vi "LiDARSteering.vi"() -> ()   [LabVIEW 2024]
uses:
  e33ea129-5426-40bd-9da2-e127971607b1.vi
  <vilib>/Instr/_visa.llb/VISA Configure Serial Port (Instr).vi
  <vilib>/Python/Open Venv Python Session.vi
panel:
  out "Input_Spd(cmd)":dbl=538.4742241275792
  in  "GoBack":bool
  in  "InputSteer(cmd)":dbl=28.559259641865033
  in  "HLV_Gear":u8
  out "PointCloud":T1(graph)=[{"appended array"=[700.0, 700.0, 3500.0, 3500.0, -3500.0, -3500.0, -700.0, -700.0, 700.0], "appended array"=[800.0, -800.0, -800.0, 5200.0, 5200.0, -800.0, -800.0, 800.0, 800.0]}, {"appended array"=[-450.0], "appended array"=[-250.0]}, {"appended array"=[-450.0, -450.0, -800.0, -800.0, 0.0, 0.0, -450.0], "appended array"=[100.0, -800.0, -800.0, 1200.0, 1200.0, 100.0, 100.0]}, {"appended array"=[800.0, 750.0, 800.0, 800.0, 800.0, 800.0, 800.0], "appended array"=[400.0, 350.0, 350.0, 300.0, 250.0, 200.0, 150.0]}, {"appended array"=[450.0, 450.0, 800.0, 800.0, 0.0, 0.0, 450.0], "appended array"=[100.0, -800.0, -800.0, 1200.0, 1200.0, 100.0, 100.0]}, {"appended array"=array[442 elements], "appended array"=array[442 elements]}, {"appended array"=[4.2861222383783204e-13, 0.0], "appended array"=[7000.0, 0.0]}, {"appended array"=[500.0, 500.0, -500.0, -500.0, 500.0], "appended array"=[100.0, 950.0, 950.0, 100.0, 100.0]}]
  in  "격자크기":dbl=50.0
  out "LidarLoop":u32=101
  in  "Ratio_Threshold":i32=4
  in  "min_samples":i32=2
  in  "eps":i32=100
  in  "Spacing":i32=100
  in  "Threshold":i32=2100
  in  "Looking Y":i32=5200
  in  "Looking X":i32=3500
  out "Anthena_Steer":i32
  out "NearSteer":dbl=28.559259641865033
  out "TooClose":bool=TRUE
  out "PythonLoop":u32=101
  in  "LiDAR":refnum<visa-resource-name>="COM5"
  out "VEstop":bool
  in  "length":dbl=1300.0
  out "read buffer":string
  out "Clustering Error":errorcluster
  out "GobackROI":cluster{i32[], i32[]}={[500, 500, -500, -500, 500], [100, 950, 950, 100, 100]}
  in  "Stop":bool
  out "TargetDerection":cluster{dbl[], dbl[]}={[4.2861222383783204e-13, 0.0], [7000.0, 0.0]}
  out "Y_arraysREAL":i32[](array[numeric])=[1650, 1650, 1650, 1650, 1650, 1650, 1650, 1650, 1700, 1700, 1700, 1700, 1700, 1700, 1700, 1700, 1700, 1700, 1700, 1750, 1700]
  out "X_arraysREAL":i32[](array[numeric])=[1000, 1050, 1100, 1150, 1200, 1250, 1300, 1350, 1350, 1400, 1450, 1500, 1550, 1600, 1650, 1700, 1750, 1800, 1850, 1850, 1900]
  out "LookingAt":cluster{i32[], i32[]}={[700, 700, 3500, 3500, -3500, -3500, -700, -700, 700], [800, -800, -800, 5200, 5200, -800, -800, 800, 800]}
  out "NearCarPointsRight":cluster{"ROI_IN_X":dbl[], "ROI_IN_Y":dbl[]}={"ROI_IN_X"=[750.0, 800.0, 800.0, 800.0, 800.0, 800.0], "ROI_IN_Y"=[350.0, 350.0, 300.0, 250.0, 200.0, 150.0]}
  out "NearCarROIRight":cluster{i32[], i32[]}={[450, 450, 800, 800, 0, 0, 450], [100, -800, -800, 1200, 1200, 100, 100]}
  out "Clustered":T2
  out "NearCarROILeft":cluster{i32[], i32[]}={[-450, -450, -800, -800, 0, 0, -450], [100, -800, -800, 1200, 1200, 100, 100]}
  out "NearCarPointsLeft":cluster{"ROI_IN_X":dbl[], "ROI_IN_Y":dbl[]}={"ROI_IN_X"=[-450.0, -550.0], "ROI_IN_Y"=[-250.0, -300.0]}
  out "Y_arrays":dbl[](array[numeric])=[1650.0, 1650.0, 1650.0, 1650.0, 1650.0, 1650.0, 1650.0, 1700.0, 1700.0, 1700.0, 1700.0, 1700.0, 1700.0, 1700.0, 1700.0, 1700.0, 1700.0, 1700.0, 1750.0, 1700.0, 1700.0, 1750.0, 1750.0, 1750.0, 1750.0, 1750.0, 1750.0, 1750.0, 1750.0, 1750.0, 1750.0, 1750.0, 1800.0, 1800.0, 1800.0, 1800.0, 1800.0, 1800.0, 1800.0, 1800.0, 1800.0, 1800.0, 1800.0, 1800.0, 1800.0, 1800.0, 1800.0, 1800.0, 1800.0, 1850.0, 1850.0, 1850.0, 350.0, 350.0, 350.0, 300.0, 250.0, 200.0, 200.0, 150.0, 150.0, 100.0, 50.0, 0.0, -50.0, -100.0, -150.0, -200.0, -250.0, -300.0, -300.0, -350.0, -400.0, -450.0, -500.0, -550.0, -600.0, -650.0, -700.0, -750.0, -800.0, -800.0, -750.0, -750.0, -700.0, -700.0, -650.0, -600.0, -550.0, -550.0, -500.0, -450.0, -400.0, -350.0, -300.0, -250.0, -200.0, -150.0, -100.0, -50.0, 0.0, 50.0, 100.0, 150.0, 200.0, 250.0, 300.0, 350.0, 400.0, 400.0, 450.0, 500.0, 550.0, 600.0, 600.0, 650.0, 650.0, 700.0, 700.0, 750.0, 750.0, 800.0, 800.0, 850.0, 850.0, 900.0, 900.0, 950.0, 950.0, 1000.0, 1000.0, 1050.0, 1050.0, 1100.0, 1100.0, 1150.0, 1150.0, 1200.0, 1200.0, 1250.0, 1250.0, 1300.0, 1300.0, 1350.0, 1400.0, 1450.0, 1500.0, 1550.0, 1600.0, 1650.0, 1700.0, 1750.0, 1800.0, 1850.0, 1900.0, 1950.0, 2000.0, 2050.0, 2100.0, 2150.0, 2200.0, 2250.0, 2300.0, 2350.0, 2400.0, 2450.0, 2500.0, 2550.0, 2600.0, 2600.0, 2650.0, 2700.0, 2750.0, 2800.0, 2850.0, 2900.0, 2950.0, 3000.0, 3050.0, 3100.0, 3150.0, 3200.0, 3250.0, 3300.0, 3350.0, 3400.0, 3450.0, 3450.0, 3500.0, 3550.0, 3600.0, 3650.0, 3700.0, 3750.0, 3800.0, 3850.0, 3900.0, 3950.0, 4000.0, 4000.0, 4100.0, 4150.0, 4200.0, 4250.0, 4300.0, 4350.0, 4400.0, 4450.0, 4500.0, 4550.0, 4600.0, 4650.0, 4700.0, 4750.0, 4800.0, 4900.0, 4950.0, 5000.0, 5050.0, 5100.0, 5150.0, 4500.0, 4500.0, 4600.0, 4550.0, 3800.0, 3700.0, 3650.0, 3600.0, 3550.0, 3500.0, 3500.0, 3450.0, 3400.0, 3350.0, 3300.0, 3250.0, 3250.0, 3200.0, 3150.0, 3200.0, 3200.0, 3200.0, 3400.0, 3450.0, 3200.0, 4700.0, 4700.0, 3700.0, 3450.0, 3400.0, 3450.0, 3500.0, 3500.0, 3450.0, 3400.0, 3400.0, 3350.0, 3300.0, 3300.0, 3250.0, 1600.0, 1600.0, 1650.0, 1600.0, 1650.0, 1735.0877192982457, -160.3448275862069, 1825.7462686567164, 5025.0, 4500.0, 4575.0, 3392.1052631578946, 3425.0, 4700.0, 3395.8333333333335, 1827.3513645224173, 1919.6150097465888, 2011.8786549707602, 2104.142300194932, 2196.4059454191033, 2288.669590643275, 2380.9332358674465, 2473.196881091618, 2565.4605263157896, 2657.7241715399614, 2749.9878167641327, 2842.251461988304, 2934.5151072124754, 3026.778752436647, 3119.042397660819, 3211.3060428849903, 3303.5696881091617, 1824.0304709141276, 1912.9732225300093, 2001.9159741458911, 2090.858725761773, 2179.801477377655, 2268.7442289935366, 2357.6869806094182, 2446.6297322253004, 2535.572483841182, 2624.5152354570637, 2713.457987072946, 2802.400738688827, 2891.343490304709, 2980.2862419205912, 3069.228993536473, 3158.1717451523546, 3247.114496768236, 3336.057248384118, 1817.938596491228, 1900.7894736842106, 1983.640350877193, 2066.4912280701756, 2149.342105263158, 2232.1929824561403, 2315.043859649123, 2397.8947368421054, 2480.745614035088, 2563.59649122807, 2646.4473684210525, 2729.2982456140353, 2812.149122807017, 2895.0, 2977.8508771929824, 3060.7017543859647, 3143.5526315789475, 3226.4035087719294, 3309.254385964912, 4515.0, 4530.0, 4545.0, 4560.0, 4407.675438596491, 4315.350877192983, 4223.026315789473, 4130.701754385965, 4038.377192982456, 3946.0526315789475, 3853.7280701754385, 3761.40350877193, 3669.078947368421, 3576.754385964912, 3484.4298245614036, 4417.307692307692, 4334.615384615385, 4251.923076923077, 4169.2307692307695, 4086.5384615384614, 4003.846153846154, 3921.153846153846, 3838.4615384615386, 3755.769230769231, 3673.076923076923, 3590.3846153846152, 3507.6923076923076, 4588.888888888889, 4602.777777777777, 4616.666666666667, 4630.555555555556, 4644.444444444444, 4658.333333333333, 4672.222222222223, 4686.111111111111, 4479.166666666667, 4383.333333333333, 4287.5, 4191.666666666667, 4095.8333333333335, 4000.0, 3904.166666666667, 3808.3333333333335, 3712.5, 3616.666666666667, 3520.8333333333335, 3403.0701754385964, 3414.035087719298, 3392.6378446115286, 3393.1704260651627, 3393.7030075187968, 3394.2355889724313, 3394.7681704260654, 3395.3007518796994, 3417.7083333333335, 3410.416666666667, 3403.125, 4684.615384615385, 4669.2307692307695, 4653.846153846154, 4638.461538461538, 4623.076923076923, 4607.692307692308, 4592.307692307692, 4576.923076923077, 4561.538461538462, 4546.153846153846, 4530.7692307692305, 4515.384615384615, 4606.8452380952385, 4513.690476190476, 4420.535714285715, 4327.380952380952, 4234.226190476191, 4141.071428571428, 4047.916666666667, 3954.761904761905, 3861.607142857143, 3768.452380952381, 3675.2976190476193, 3582.1428571428573, 3488.9880952380954, 3486.538461538462, 3577.24358974359, 3667.9487179487182, 3758.653846153846, 3849.3589743589746, 3940.0641025641025, 4030.769230769231, 4121.474358974359, 4212.179487179487, 4302.884615384615, 4393.589743589744, 4484.294871794872]
  out "X_arrays":dbl[](array[numeric])=[1050.0, 1100.0, 1150.0, 1200.0, 1250.0, 1300.0, 1350.0, 1350.0, 1400.0, 1450.0, 1500.0, 1550.0, 1600.0, 1650.0, 1700.0, 1750.0, 1800.0, 1850.0, 1850.0, 1900.0, 1950.0, 2000.0, 2050.0, 2100.0, 2150.0, 2200.0, 2250.0, 2300.0, 2350.0, 2400.0, 2450.0, 2500.0, 2500.0, 2550.0, 2600.0, 2650.0, 2700.0, 2750.0, 2800.0, 2850.0, 2900.0, 2950.0, 3000.0, 3050.0, 3100.0, 3150.0, 3200.0, 3250.0, 3300.0, 3350.0, 3400.0, 3450.0, 750.0, 800.0, 850.0, 800.0, 800.0, 800.0, 850.0, 800.0, 850.0, 850.0, 850.0, 850.0, 850.0, 850.0, 850.0, 850.0, 850.0, 850.0, 900.0, 900.0, 900.0, 900.0, 900.0, 900.0, 900.0, 900.0, 900.0, 900.0, 900.0, -2250.0, -2250.0, -2300.0, -2300.0, -2250.0, -2300.0, -2300.0, -2300.0, -2350.0, -2300.0, -2300.0, -2300.0, -2300.0, -2300.0, -2300.0, -2300.0, -2300.0, -2300.0, -2300.0, -2300.0, -2300.0, -2300.0, -2300.0, -2300.0, -2300.0, -2300.0, -2300.0, -2250.0, -2300.0, -2300.0, -2300.0, -2300.0, -2300.0, -2250.0, -2250.0, -2300.0, -2250.0, -2300.0, -2300.0, -2250.0, -2300.0, -2250.0, -2300.0, -2250.0, -2300.0, -2250.0, -2250.0, -2300.0, -2300.0, -2250.0, -2250.0, -2300.0, -2250.0, -2300.0, -2250.0, -2300.0, -2250.0, -2300.0, -2300.0, -2250.0, -2300.0, -2250.0, -2250.0, -2250.0, -2250.0, -2250.0, -2250.0, -2250.0, -2250.0, -2250.0, -2250.0, -2250.0, -2250.0, -2250.0, -2250.0, -2250.0, -2250.0, -2250.0, -2250.0, -2250.0, -2250.0, -2250.0, -2250.0, -2250.0, -2250.0, -2250.0, -2250.0, -2250.0, -2300.0, -2300.0, -2300.0, -2300.0, -2300.0, -2300.0, -2300.0, -2300.0, -2300.0, -2300.0, -2300.0, -2300.0, -2300.0, -2300.0, -2300.0, -2300.0, -2300.0, -2300.0, -2350.0, -2350.0, -2350.0, -2350.0, -2350.0, -2350.0, -2350.0, -2350.0, -2350.0, -2350.0, -2350.0, -2350.0, -2400.0, -2400.0, -2400.0, -2400.0, -2400.0, -2400.0, -2400.0, -2400.0, -2400.0, -2400.0, -2400.0, -2400.0, -2400.0, -2400.0, -2400.0, -2400.0, -2450.0, -2450.0, -2450.0, -2450.0, -2450.0, -2450.0, 650.0, 700.0, 1100.0, 1150.0, 950.0, 950.0, 950.0, 950.0, 950.0, 950.0, 1000.0, 1000.0, 1000.0, 1000.0, 1000.0, 1000.0, 1050.0, 1050.0, 1050.0, 1100.0, 1150.0, 1200.0, 1300.0, 1350.0, 1250.0, 1900.0, 1950.0, 1600.0, 1500.0, 1550.0, 1600.0, 1600.0, 1650.0, 1650.0, 1650.0, 1700.0, 1650.0, 1650.0, 1700.0, 1700.0, 900.0, 950.0, 950.0, 1000.0, 1000.0, 2118.4210526315787, 856.8965517241379, -2300.0, -2450.0, 675.0, 1125.0, 1028.9473684210527, 1325.0, 1925.0, 1633.3333333333333, 2091.4717348927875, 2064.522417153996, 2037.5730994152045, 2010.623781676413, 1983.6744639376216, 1956.7251461988303, 1929.7758284600388, 1902.8265107212474, 1875.877192982456, 1848.9278752436646, 1821.9785575048732, 1795.029239766082, 1768.0799220272904, 1741.130604288499, 1714.1812865497075, 1687.231968810916, 1660.2826510721247, 2076.6620498614957, 2034.9030470914126, 1993.1440443213294, 1951.3850415512463, 1909.6260387811633, 1867.8670360110802, 1826.108033240997, 1784.349030470914, 1742.590027700831, 1700.8310249307478, 1659.0720221606648, 1617.3130193905818, 1575.5540166204987, 1533.7950138504154, 1492.0360110803324, 1450.2770083102494, 1408.5180055401663, 1366.759002770083, 2063.9473684210525, 2009.4736842105262, 1954.9999999999998, 1900.5263157894735, 1846.0526315789473, 1791.5789473684208, 1737.1052631578946, 1682.6315789473683, 1628.157894736842, 1573.6842105263158, 1519.2105263157894, 1464.736842105263, 1410.2631578947367, 1355.7894736842104, 1301.3157894736842, 1246.842105263158, 1192.3684210526317, 1137.8947368421054, 1083.421052631579, 765.0, 855.0, 945.0, 1035.0, 704.4956140350878, 733.9912280701755, 763.4868421052631, 792.9824561403509, 822.4780701754387, 851.9736842105264, 881.469298245614, 910.9649122807018, 940.4605263157896, 969.9561403508773, 999.4517543859649, 725.0, 775.0, 825.0, 875.0, 925.0, 975.0, 1025.0, 1075.0, 1125.0, 1175.0, 1225.0, 1275.0, 1213.888888888889, 1302.7777777777778, 1391.6666666666665, 1480.5555555555557, 1569.4444444444443, 1658.3333333333333, 1747.2222222222222, 1836.111111111111, 1141.6666666666667, 1158.3333333333333, 1175.0, 1191.6666666666667, 1208.3333333333333, 1225.0, 1241.6666666666667, 1258.3333333333333, 1275.0, 1291.6666666666667, 1308.3333333333333, 1127.6315789473686, 1226.3157894736842, 1115.2882205513786, 1201.6290726817042, 1287.96992481203, 1374.310776942356, 1460.6516290726815, 1546.9924812030074, 1402.0833333333333, 1479.1666666666665, 1556.25, 1828.8461538461538, 1732.6923076923076, 1636.5384615384614, 1540.3846153846152, 1444.2307692307693, 1348.076923076923, 1251.9230769230767, 1155.7692307692307, 1059.6153846153848, 963.4615384615385, 867.3076923076922, 771.1538461538462, 1904.1666666666667, 1883.3333333333333, 1862.5, 1841.6666666666667, 1820.8333333333333, 1800.0, 1779.1666666666665, 1758.3333333333333, 1737.5, 1716.6666666666665, 1695.8333333333333, 1675.0, 1654.1666666666665, 1594.230769230769, 1555.128205128205, 1516.0256410256409, 1476.923076923077, 1437.8205128205127, 1398.7179487179487, 1359.6153846153845, 1320.5128205128203, 1281.4102564102564, 1242.3076923076924, 1203.2051282051282, 1164.102564102564]
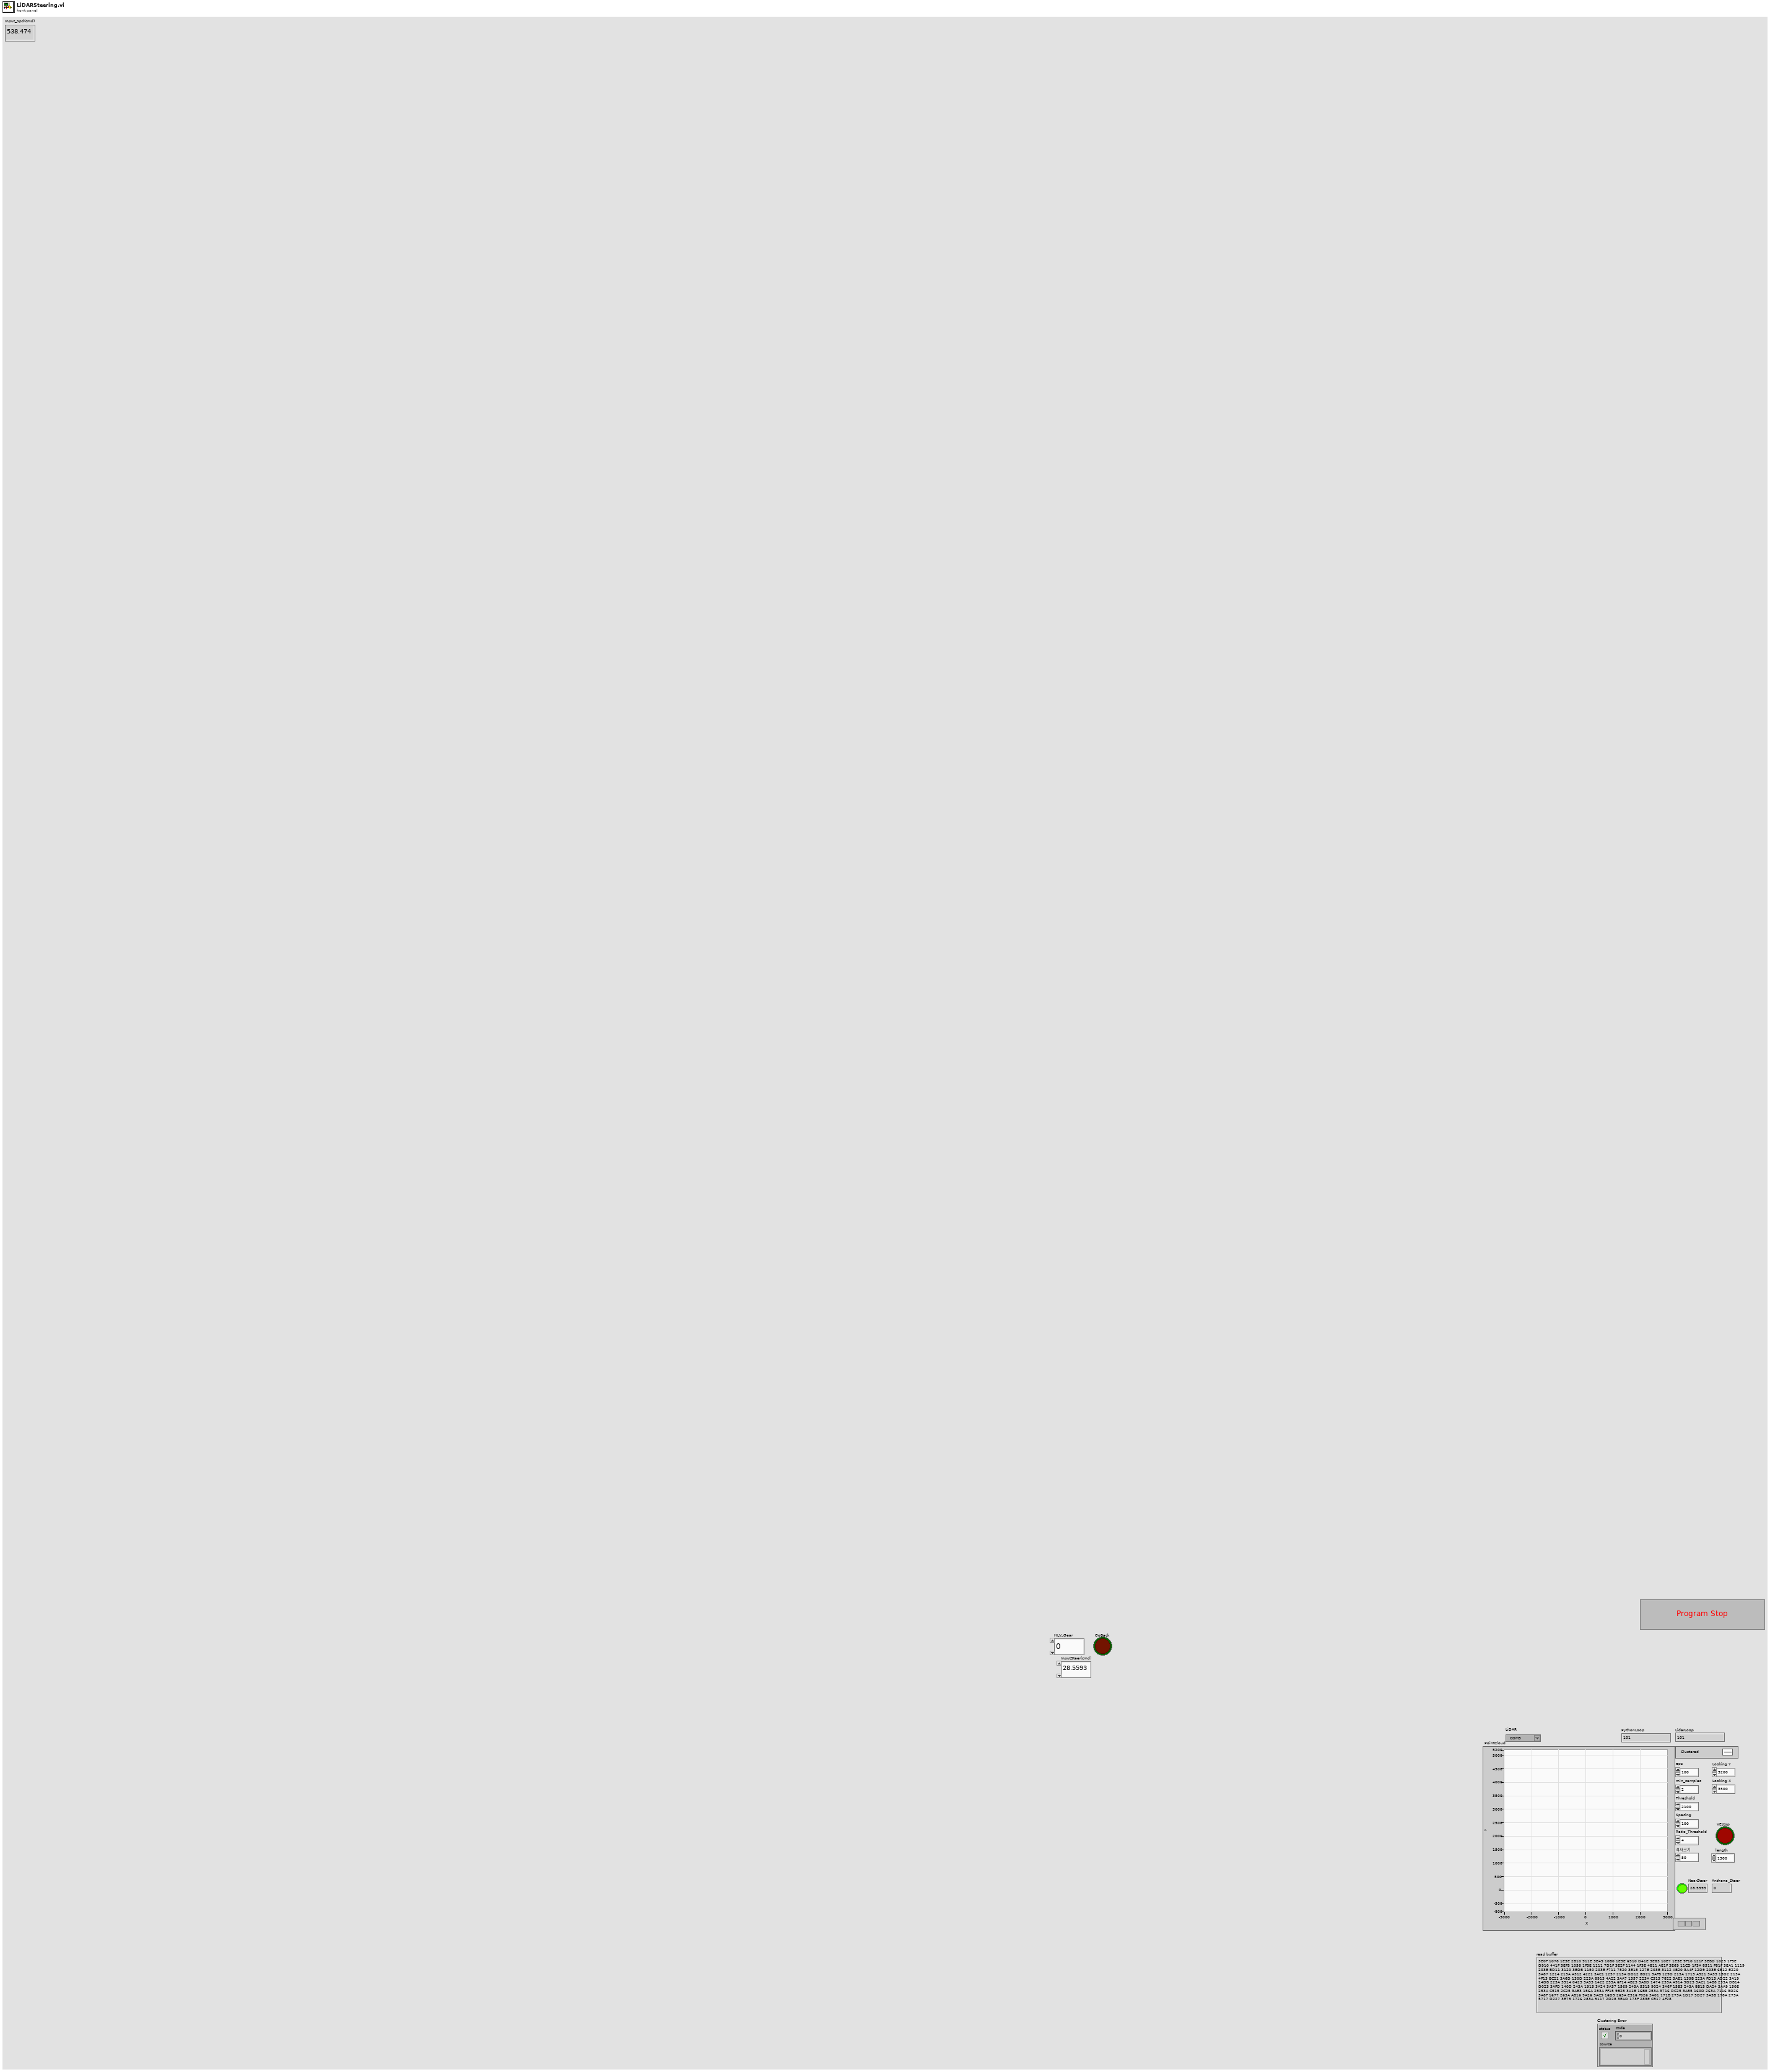
[diagram p1: front panel]
types:
  T1 = cluster{"appended array":dbl[], "appended array":dbl[]}[]
  T2 = cluster{"appended array":dbl[], "appended array":dbl[]}
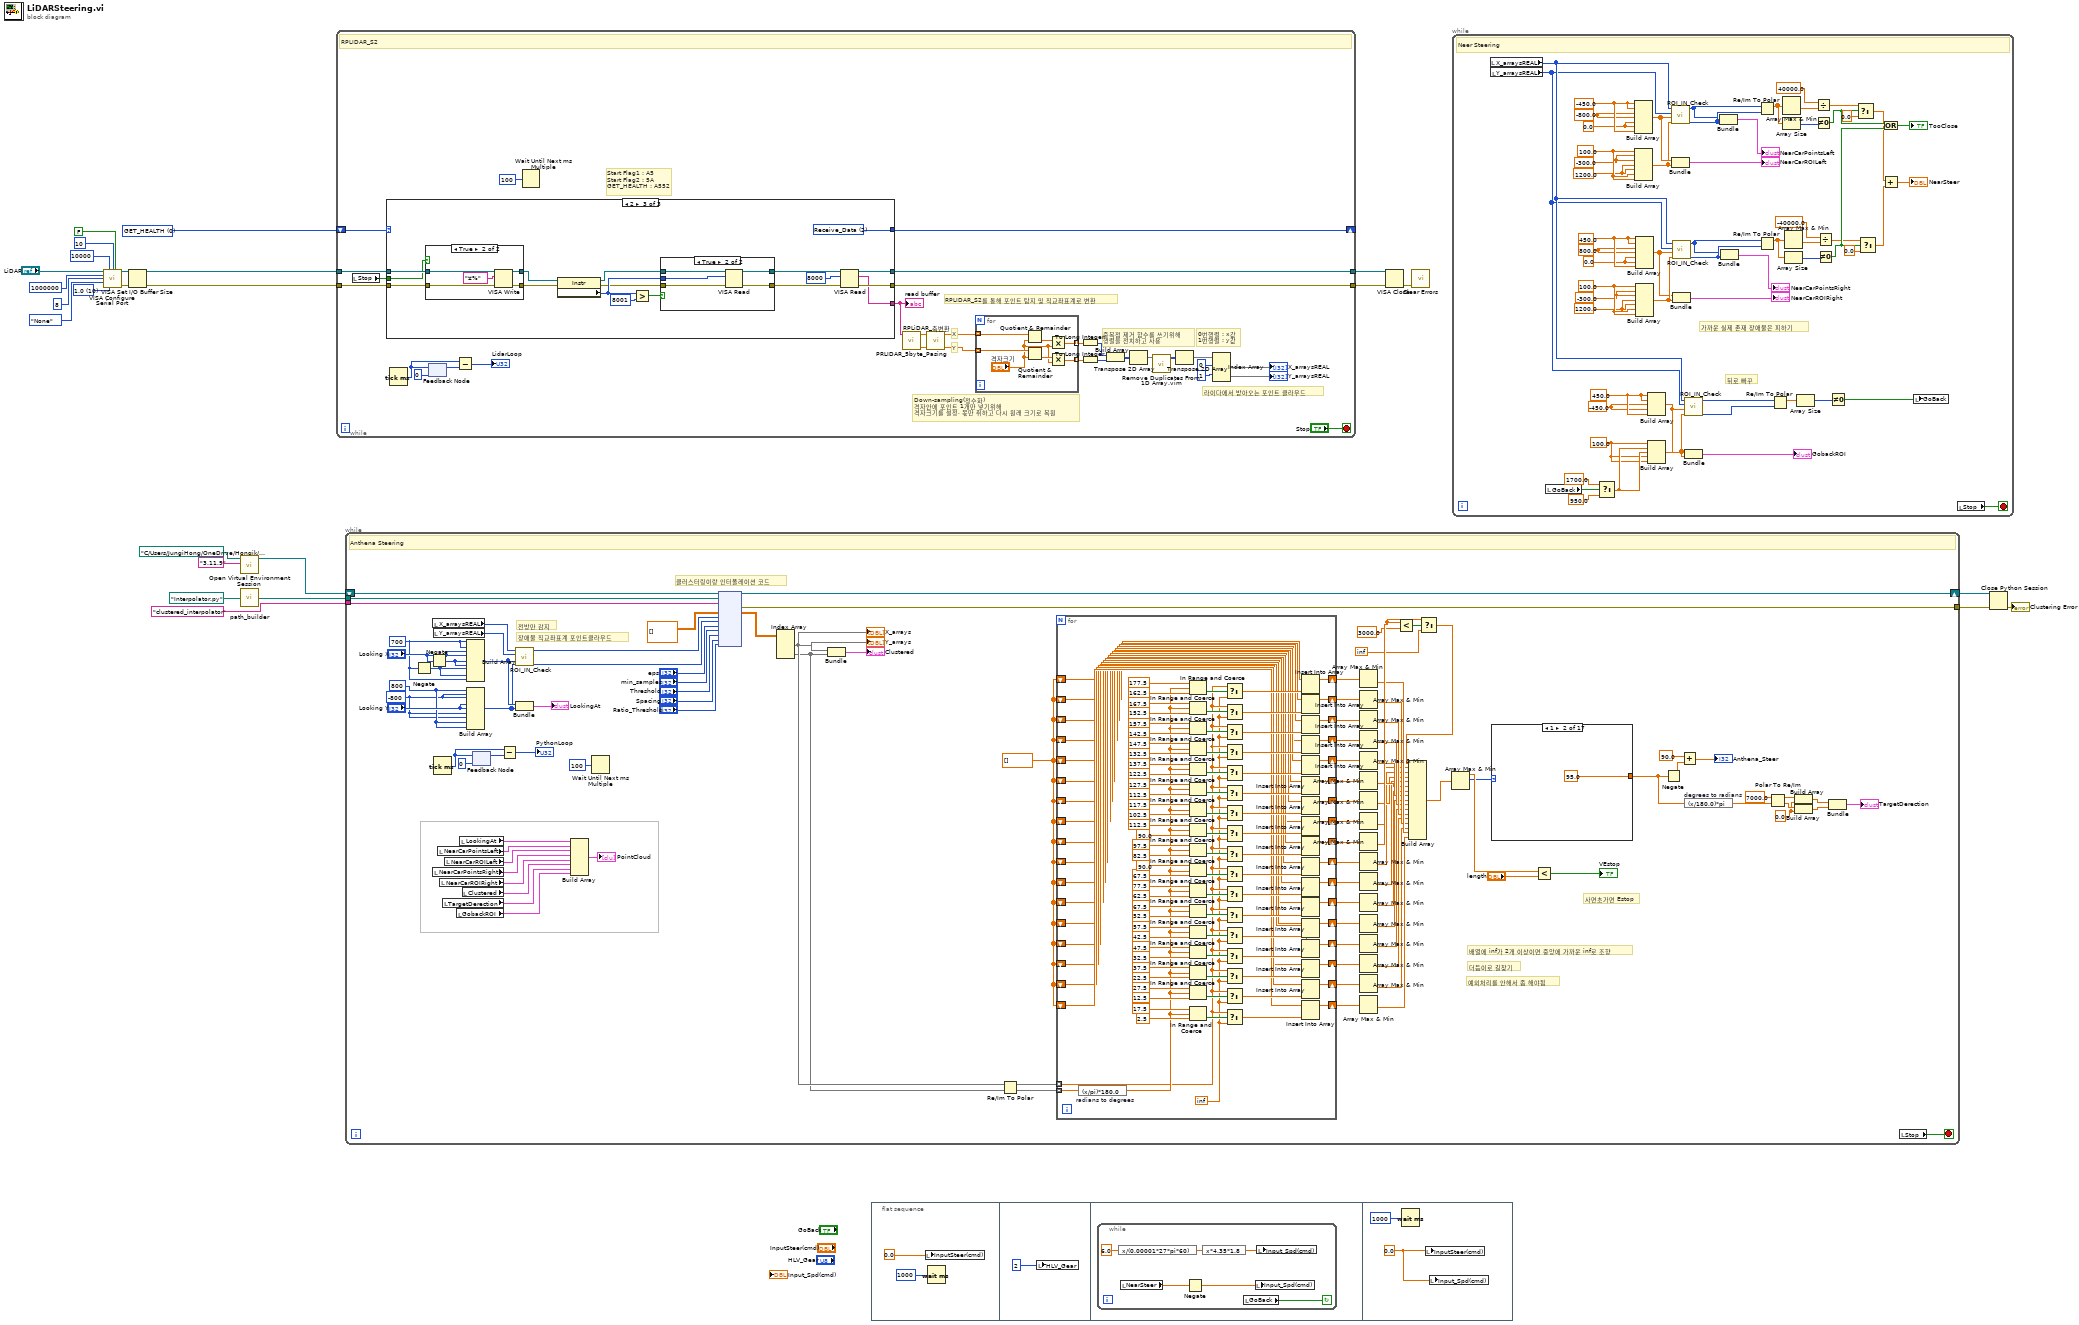
[diagram p0: block diagram]
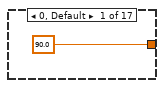
[diagram p2: hidden frame]
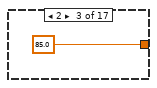
[diagram p3: hidden frame]
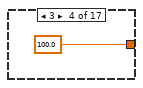
[diagram p4: hidden frame]
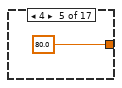
[diagram p5: hidden frame]
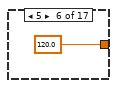
[diagram p6: hidden frame]
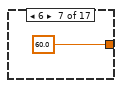
[diagram p7: hidden frame]
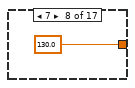
[diagram p8: hidden frame]
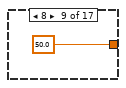
[diagram p9: hidden frame]
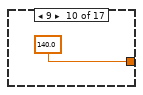
[diagram p10: hidden frame]
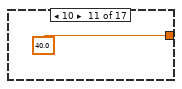
[diagram p11: hidden frame]
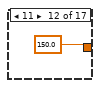
[diagram p12: hidden frame]
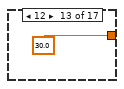
[diagram p13: hidden frame]
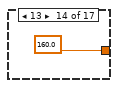
[diagram p14: hidden frame]
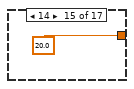
[diagram p15: hidden frame]
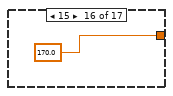
[diagram p16: hidden frame]
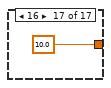
[diagram p17: hidden frame]
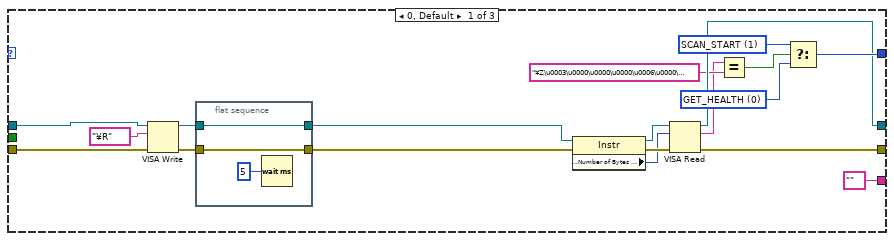
[diagram p18: hidden frame]
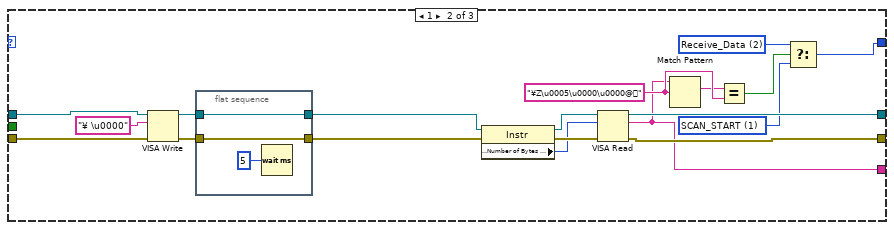
[diagram p19: hidden frame]
diagram:
  w11 = u16 10 items=["1.0"=10, "1.5"=15, "2.0"=20] ("stop bits (10: 1 bit)")
  w13 = u16 0 items=["GET_HEALTH", "SCAN_START", "Receive_Data"]
  n1 = call-poly "VISA Configure Serial Port"("VISA resource name"="LiDAR", "timeout (10sec)"=u32 10000, "termination char\n(0xA = '\\n' = LF)"=u8 10 ("termination char\n(0xA = '\\n' = LF)"), "Enable Termination\nChar (T)"=FALSE ("Enable Termination\nChar (T)"), "baud rate (9600)"=u32 1000000, "data bits (8)"=u16 8, "parity (0:none)"=enum16{"None", "Odd", "Even", "Mark", "Space"}."None", "stop bits (10: 1 bit)"=w11) -> ("VISA resource name out"=w20:refnum<visa-resource-name>, "error out"=w19:errorcluster)  [unwired: 6 in]
  n2 = VISA Set I/O Buffer Size(VISA resource name=w20, error in (no error)=w19) -> (VISA resource name out=w15:refnum<visa-resource-name>, error out=w14:errorcluster)  [unwired: 2 in]
  n3 = call-poly <vilib>:"Open Virtual Environment Session.vi"("Python version"="3.11.9", "Env path"=path "C:/Users/JungiHong/OneDrive/Hongik/HI-RACE/2026-01/.venv" ("Name")) -> ("session out"=w2:refnum<k35>)  [unwired: 8 in, 1 out]
  n4 = call "path_builder.vi"("Name"=path "Interpolator.py") -> ("appended path"=w6:path)
  n5 = while {
    tunnel: [w45] -> w24
    tunnel: [w46] -> w23
    tunnel: w15 -> [w54]
    tunnel: w14 -> [w53]
    shift-right: [w52] -> _
    shift-left: w13 -> [w55]
    stop <- "Stop" stop-if-true
    # "라이다에서 받아오는 포인트 클라우드"
    # "RPLIDAR_S2를 통해 포인트 탐지 및 직교좌표계로 변환"
    # "Start Flag1 : A5\nStart Flag2 : 5A \nGET_HEALTH : A552"
    # "0번행렬 : x값\n1번행렬 : y값"
    # "중복점 제거 함수를 쓰기위해\n행렬을 전치하고 사용"
    # "Down-sampling(정수화)\n격자안에 포인트 1개만 넣기위해\n격자크기를 설정, 몫만 취하고 다시 원래 크기로 복원"
    # "Y"
    # "X"
    # "RPLIDAR_S2"
    n6 = local read "Stop"() -> (w51:bool)
    n7 = case shown="2" w55 {
      tunnel: w54 -> [w80 w98 w121]
      tunnel: w53 -> [w79 w97 w120]
      tunnel: [w81 w94 w107] -> w52
      tunnel: [w70 w95 w123] -> w46
      tunnel: [w69 w96 w122] -> w45
      tunnel: w51 -> [_ _ w119]
      tunnel: ["" ("read buffer") w92 w118] -> w30
      frame 0, Default {
        w63 = u16 0 items=["GET_HEALTH", "SCAN_START", "Receive_Data"]
        w64 = u16 1 items=["GET_HEALTH", "SCAN_START", "Receive_Data"]
        n8 = VISA Write(VISA resource name=w80, write buffer="¥R", error in (no error)=w79) -> (VISA resource name out=w74:refnum<visa-resource-name>, error out=w73:errorcluster)  [unwired: 1 out]
        n9 = flat-sequence {
          tunnel: w74 -> [w83]
          tunnel: w73 -> [w82]
          tunnel: [w83] -> w72
          tunnel: [w82] -> w71
          frame #0 {
            n10 = Wait (ms)(milliseconds to wait=u32 5 ("대기 시간 (ms)")) -> ()  [unwired: 1 out]
          }
        }
        n11 = property class="Instr"(reference=w72, error in=w71) -> (reference out=w77:refnum<visa-resource-name>, error out=w76:errorcluster, "Serial Settings:Number of Bytes at Serial Port"=w75:u32)
        n12 = VISA Read(VISA resource name=w77, byte count=w75, error in (no error)=w76) -> (VISA resource name out=w69:refnum<visa-resource-name>, read buffer=w66:string, error out=w70:errorcluster)  [unwired: 1 out]
        n13 = Equal?(x=w66, y="¥Z\u0003\u0000\u0000\u0000\u0006\u0000\u0000\u0000") -> (x = y?=w67:bool)
        n14 = Select(t=w64, s=w67, f=w63) -> (s? t:f=w81:u16)
      }
      frame 1 {
        w85 = u16 2 items=["GET_HEALTH", "SCAN_START", "Receive_Data"]
        w86 = u16 1 items=["GET_HEALTH", "SCAN_START", "Receive_Data"]
        w99 = "¥Z\u0005\u0000\u0000@"
        n15 = VISA Write(VISA resource name=w98, write buffer="¥ \u0000", error in (no error)=w97) -> (VISA resource name out=w101:refnum<visa-resource-name>, error out=w102:errorcluster)  [unwired: 1 out]
        n16 = flat-sequence {
          tunnel: w101 -> [w105]
          tunnel: w102 -> [w104]
          tunnel: [w105] -> w88
          tunnel: [w104] -> w87
          frame #0 {
            n17 = Wait (ms)(milliseconds to wait=u32 5 ("대기 시간 (ms)")) -> ()  [unwired: 1 out]
          }
        }
        n18 = property class="Instr"(reference=w88, error in=w87) -> (reference out=w91:refnum<visa-resource-name>, error out=w90:errorcluster, "Serial Settings:Number of Bytes at Serial Port"=w89:u32)
        n19 = VISA Read(VISA resource name=w91, byte count=w89, error in (no error)=w90) -> (VISA resource name out=w96:refnum<visa-resource-name>, read buffer=w92:string, error out=w95:errorcluster)  [unwired: 1 out]
        n20 = Match Pattern(string=w92, regular expression=w99) -> (match substring=w93:string)  [unwired: 1 in, 3 out]
        n21 = Equal?(x=w93, y=w99) -> (x = y?=w103:bool)
        n22 = Select(t=w85, s=w103, f=w86) -> (s? t:f=w94:u16)
      }
      frame 2 {
        w107 = u16 2 items=["GET_HEALTH", "SCAN_START", "Receive_Data"]
        n23 = case shown="True" w119 {
          tunnel: w121 -> [w132 w136]
          tunnel: w120 -> [w131 w135]
          tunnel: [w132 w134] -> w117
          tunnel: [w131 w133] -> w116
          frame False {
          }
          frame True {
            n24 = VISA Write(VISA resource name=w136, write buffer="¥%", error in (no error)=w135) -> (VISA resource name out=w134:refnum<visa-resource-name>, error out=w133:errorcluster)  [unwired: 1 out]
          }
        }
        n25 = property class="Instr"(reference=w117, error in=w116) -> (reference out=w112:refnum<visa-resource-name>, error out=w111:errorcluster, "Serial Settings:Number of Bytes at Serial Port"=w113:u32)
        n26 = Greater?(x=w113, y=u32 8001) -> (0:w115:bool)
        n27 = case shown="True" w115 {
          tunnel: w112 -> [w125 w130]
          tunnel: w113 -> [_ w129]
          tunnel: w111 -> [w124 w128]
          tunnel: [w125 w127] -> w110
          tunnel: [w124 w126] -> w109
          frame False {
          }
          frame True {
            n28 = VISA Read(VISA resource name=w130, byte count=w129, error in (no error)=w128) -> (VISA resource name out=w127:refnum<visa-resource-name>, error out=w126:errorcluster)  [unwired: 2 out]
          }
        }
        n29 = VISA Read(VISA resource name=w110, byte count=u32 8000, error in (no error)=w109) -> (VISA resource name out=w122:refnum<visa-resource-name>, read buffer=w118:string, error out=w123:errorcluster)  [unwired: 1 out]
      }
    }
    "read buffer" <- w30
    n30 = Tick Count (ms)() -> (millisecond timer value=w50:u32)
    n31 = feedback #1(u32 0 ("millisecond timer value")) -> (w49:u32)
    n32 = feedback-in #1(w50) -> ()
    n33 = Subtract(x=w50, y=w49) -> (x-y=→"LidarLoop":u32)
    n34 = Wait Until Next ms Multiple(millisecond multiple=u32 100) -> ()  [unwired: 1 out]
    n35 = call "PRLIDAR_5byte_Pasing.vi"("RPLIDAR_Data"=w30) -> ("Theta(deg)"=w33:dbl[], "Distance(mm)"=w34:dbl[])  [unwired: 9 in]
    n36 = call "RPLiDAR_축변환.vi"("Distance(mm)"=w33, "Theta(deg)"=w34) -> ("Y"=w31:dbl[], "X"=w32:dbl[])  [unwired: 8 in]
    n37 = for {
      tunnel: w32 -> [w62] mode=indexing
      tunnel: w31 -> [w61] mode=indexing
      tunnel: [w58] -> w43 mode=indexing
      tunnel: [w57] -> w44 mode=indexing
      n38 = Quotient & Remainder(x=w62, y="격자크기") -> (floor(x/y)=w60:dbl)  [unwired: 1 out]
      n39 = Quotient & Remainder(x=w61, y="격자크기") -> (floor(x/y)=w59:dbl)  [unwired: 1 out]
      n40 = Multiply(x=w60, y="격자크기") -> (x*y=w58:dbl)
      n41 = Multiply(x=w59, y="격자크기") -> (x*y=w57:dbl)
    }
    n42 = To Long Integer(number=w43) -> (32bit integer=w38:i32[])
    n43 = To Long Integer(number=w44) -> (32bit integer=w37:i32[])
    n44 = Build Array(w38, w37) -> (w39:i32[][])
    n45 = Transpose 2D Array(2D array=w39) -> (transposed array=w35:i32[][])
    n46 = call "Remove Duplicates From 1D Array.vim"("array"=w35) -> ("array with duplicates removed"=w36:i32[][])  [unwired: 10 in]
    n47 = Transpose 2D Array(2D array=w36) -> (transposed array=w40:i32[][])
    n48 = Index Array(array=w40, index (row) #1=0 ("index (row)"), index (row) #2=1 ("index (row)")) -> (element #1=→"X_arraysREAL":i32[], element #2=→"Y_arraysREAL":i32[])  [unwired: 2 in]
  }
  n49 = while {
    tunnel: [w239] -> w10
    tunnel: "clustered_interpolator" ("function name") -> [w237]
    tunnel: w6 -> [w236]
    shift-right: [w238] -> w9
    shift-left: w2 -> [w235]
    stop <- w147 stop-if-true
    w150 = dbl[] []
    w152 = 0.0 ("r")
    w212 = -800
    w213 = 800
    w214 = 700
    # "사면초가면 Estop"
    # "배열에 inf가 2개 이상이면 중앙에 가까운 inf로 조향"
    # "예외처리를 안해서 좀 해야됨"
    # "더듬이로 길찾기"
    # "전방만 감지"
    # "장애물 직교좌표계 포인트클라우드"
    # "클러스터링이랑 인터폴레이션 코드"
    # "Anthena Steering"
    n50 = Negate(x=w214) -> (-x=w217:i32)
    n51 = Negate(x="Looking X") -> (-x=w218:i32)
    n52 = local read "X_arraysREAL"() -> (w211:i32[])
    n53 = local read "NearCarPointsRight"() -> (w144:cluster{"ROI_IN_X":dbl[], "ROI_IN_Y":dbl[]})
    n54 = local read "Y_arraysREAL"() -> (w210:i32[])
    n55 = Tick Count (ms)() -> (millisecond timer value=w222:u32)
    n56 = local read "NearCarPointsLeft"() -> (w141:cluster{"ROI_IN_X":dbl[], "ROI_IN_Y":dbl[]})
    n57 = local read "NearCarROIRight"() -> (w145:cluster{i32[], i32[]})
    n58 = local read "TargetDerection"() -> (w139:cluster{dbl[], dbl[]})
    n59 = local read "NearCarROILeft"() -> (w142:cluster{i32[], i32[]})
    n60 = local read "GobackROI"() -> (w138:cluster{i32[], i32[]})
    n61 = local read "LookingAt"() -> (w140:cluster{i32[], i32[]})
    n62 = local read "Clustered"() -> (w146:T2)
    n63 = Build Array(w214, w214, "Looking X", "Looking X", w218, w218, w217, w217, w214) -> (w220:i32[])
    n64 = Build Array(w213, w212, w212, "Looking Y", "Looking Y", w212, w212, w213, w213) -> (w219:i32[])
    n65 = feedback #2(u32 0 ("millisecond timer value")) -> (w223:u32)
    n66 = feedback-in #2(w222) -> ()
    n67 = Subtract(x=w222, y=w223) -> (x-y=→"PythonLoop":u32)
    n68 = call "ROI_IN_Check.vi"("도형Y좌표"=w219, "도형X좌표"=w220, "LiDAR_Y"=w210, "LiDAR_X"=w211) -> ("ROI_IN_Y"=w208:i32[], "ROI_IN_X"=w209:i32[])  [unwired: 6 in]
    n69 = Bundle(w220, w219) -> (→"LookingAt":cluster{i32[], i32[]})  [unwired: 1 in]
    n70 = Build Array(w140, w141, w142, w144, w145, w146, w139, w138) -> (→"PointCloud":T1)
    n71 = Wait Until Next ms Multiple(millisecond multiple=u32 100) -> ()  [unwired: 1 out]
    n72 = node(w235, w236, w237, dbl[][] [] ("appended array"), w209, w208, "eps", "min_samples", "Threshold", "Spacing", "Ratio_Threshold") -> (w238:refnum<k35>, w239:errorcluster, w234:dbl[][])  [unwired: 8 in, 2 out]
    n73 = Index Array(array=w234) -> (element #1=w149:dbl[], element #2=w148:dbl[])  [unwired: 4 in]
    "X_arrays" <- w149
    "Y_arrays" <- w148
    n74 = Bundle("appended array"=w149, "appended array"=w148) -> (→"Clustered":T2)  [unwired: 1 in]
    n75 = Re/Im To Polar(2:w148, 3:w149) -> (0:w156:dbl[], 1:w157:dbl[])
    n76 = for {
      tunnel: w156 -> [w362] mode=indexing
      tunnel: w157 -> [w284] mode=indexing
      shift-right: [w329] -> w158
      shift-left: w150 -> [w261]
      shift-right: [w328] -> w159
      shift-left: w150 -> [w262]
      shift-right: [w327] -> w160
      shift-left: w150 -> [w263]
      shift-right: [w326] -> w161
      shift-left: w150 -> [w264]
      shift-right: [w325] -> w162
      shift-left: w150 -> [w265]
      shift-right: [w324] -> w163
      shift-left: w150 -> [w266]
      shift-right: [w323] -> w164
      shift-left: w150 -> [w267]
      shift-right: [w322] -> w165
      shift-left: w150 -> [w268]
      shift-right: [w318] -> w171
      shift-left: w150 -> [w269]
      shift-right: [w282] -> w186
      shift-left: w150 -> [w270]
      shift-right: [w281] -> w187
      shift-left: w150 -> [w271]
      shift-right: [w280] -> w188
      shift-left: w150 -> [w272]
      shift-right: [w279] -> w189
      shift-left: w150 -> [w273]
      shift-right: [w275] -> w193
      shift-left: w150 -> [w257]
      shift-right: [w276] -> w192
      shift-left: w150 -> [w258]
      shift-right: [w277] -> w191
      shift-left: w150 -> [w259]
      shift-right: [w278] -> w190
      shift-left: w150 -> [w260]
      w283 = inf
      n77 = expression code="(x/pi)*180.0" "radians to degrees"(w362) -> (w302:dbl)
      n78 = In Range and Coerce(upper limit=177.5, x=w302, lower limit=162.5) -> (In Range?=w289:bool)  [unwired: 1 out]
      n79 = In Range and Coerce(upper limit=167.5, x=w302, lower limit=152.5 ("upper limit")) -> (In Range?=w290:bool)  [unwired: 1 out]
      n80 = In Range and Coerce(upper limit=157.5 ("lower limit"), x=w302, lower limit=142.5 ("upper limit")) -> (In Range?=w291:bool)  [unwired: 1 out]
      n81 = In Range and Coerce(upper limit=147.5 ("lower limit"), x=w302, lower limit=132.5 ("upper limit")) -> (In Range?=w292:bool)  [unwired: 1 out]
      n82 = In Range and Coerce(upper limit=137.5, x=w302, lower limit=122.5) -> (In Range?=w343:bool)  [unwired: 1 out]
      n83 = In Range and Coerce(upper limit=127.5, x=w302, lower limit=112.5) -> (In Range?=w345:bool)  [unwired: 1 out]
      n84 = In Range and Coerce(upper limit=117.5, x=w302, lower limit=102.5) -> (In Range?=w341:bool)  [unwired: 1 out]
      n85 = In Range and Coerce(upper limit=112.5, x=w302, lower limit=90.0) -> (In Range?=w340:bool)  [unwired: 1 out]
      n86 = In Range and Coerce(upper limit=97.5, x=w302, lower limit=82.5) -> (In Range?=w339:bool)  [unwired: 1 out]
      n87 = In Range and Coerce(upper limit=90.0, x=w302, lower limit=67.5) -> (In Range?=w338:bool)  [unwired: 1 out]
      n88 = In Range and Coerce(upper limit=77.5, x=w302, lower limit=62.5) -> (In Range?=w337:bool)  [unwired: 1 out]
      n89 = In Range and Coerce(upper limit=67.5, x=w302, lower limit=52.5) -> (In Range?=w336:bool)  [unwired: 1 out]
      n90 = In Range and Coerce(upper limit=57.5, x=w302, lower limit=42.5) -> (In Range?=w321:bool)  [unwired: 1 out]
      n91 = In Range and Coerce(upper limit=47.5, x=w302, lower limit=32.5) -> (In Range?=w300:bool)  [unwired: 1 out]
      n92 = In Range and Coerce(upper limit=37.5, x=w302, lower limit=22.5) -> (In Range?=w299:bool)  [unwired: 1 out]
      n93 = In Range and Coerce(upper limit=27.5, x=w302, lower limit=12.5) -> (In Range?=w298:bool)  [unwired: 1 out]
      n94 = In Range and Coerce(upper limit=17.5, x=w302, lower limit=2.5) -> (In Range?=w297:bool)  [unwired: 1 out]
      n95 = Select(t=w284, s=w289, f=w283) -> (s? t:f=w288:dbl)
      n96 = Select(t=w284, s=w290, f=w283) -> (s? t:f=w287:dbl)
      n97 = Select(t=w284, s=w291, f=w283) -> (s? t:f=w286:dbl)
      n98 = Select(t=w284, s=w292, f=w283) -> (s? t:f=w285:dbl)
      n99 = Select(t=w284, s=w343, f=w283) -> (s? t:f=w342:dbl)
      n100 = Select(t=w284, s=w345, f=w283) -> (s? t:f=w344:dbl)
      n101 = Select(t=w284, s=w341, f=w283) -> (s? t:f=w330:dbl)
      n102 = Select(t=w284, s=w340, f=w283) -> (s? t:f=w331:dbl)
      n103 = Select(t=w284, s=w339, f=w283) -> (s? t:f=w332:dbl)
      n104 = Select(t=w284, s=w338, f=w283) -> (s? t:f=w333:dbl)
      n105 = Select(t=w284, s=w337, f=w283) -> (s? t:f=w334:dbl)
      n106 = Select(t=w284, s=w336, f=w283) -> (s? t:f=w335:dbl)
      n107 = Select(t=w284, s=w321, f=w283) -> (s? t:f=w301:dbl)
      n108 = Select(t=w284, s=w300, f=w283) -> (s? t:f=w296:dbl)
      n109 = Select(t=w284, s=w299, f=w283) -> (s? t:f=w295:dbl)
      n110 = Select(t=w284, s=w298, f=w283) -> (s? t:f=w294:dbl)
      n111 = Select(t=w284, s=w297, f=w283) -> (s? t:f=w293:dbl)
      n112 = Insert Into Array(array=w257, new element=w288) -> (w275:dbl[])  [unwired: 1 in]
      n113 = Insert Into Array(array=w258, new element=w287) -> (w276:dbl[])  [unwired: 1 in]
      n114 = Insert Into Array(array=w259, new element=w286) -> (w277:dbl[])  [unwired: 1 in]
      n115 = Insert Into Array(array=w260, new element=w285) -> (w278:dbl[])  [unwired: 1 in]
      n116 = Insert Into Array(array=w261, new element=w342) -> (w329:dbl[])  [unwired: 1 in]
      n117 = Insert Into Array(array=w262, new element=w344) -> (w328:dbl[])  [unwired: 1 in]
      n118 = Insert Into Array(array=w263, new element=w330) -> (w327:dbl[])  [unwired: 1 in]
      n119 = Insert Into Array(array=w264, new element=w331) -> (w326:dbl[])  [unwired: 1 in]
      n120 = Insert Into Array(array=w265, new element=w332) -> (w325:dbl[])  [unwired: 1 in]
      n121 = Insert Into Array(array=w266, new element=w333) -> (w324:dbl[])  [unwired: 1 in]
      n122 = Insert Into Array(array=w267, new element=w334) -> (w323:dbl[])  [unwired: 1 in]
      n123 = Insert Into Array(array=w268, new element=w335) -> (w322:dbl[])  [unwired: 1 in]
      n124 = Insert Into Array(array=w269, new element=w301) -> (w318:dbl[])  [unwired: 1 in]
      n125 = Insert Into Array(array=w270, new element=w296) -> (w282:dbl[])  [unwired: 1 in]
      n126 = Insert Into Array(array=w271, new element=w295) -> (w281:dbl[])  [unwired: 1 in]
      n127 = Insert Into Array(array=w272, new element=w294) -> (w280:dbl[])  [unwired: 1 in]
      n128 = Insert Into Array(array=w273, new element=w293) -> (w279:dbl[])  [unwired: 1 in]
    }
    n129 = Array Max & Min(array=w193) -> (min value=w200:dbl)  [unwired: 3 out]
    n130 = Array Max & Min(array=w192) -> (min value=w198:dbl)  [unwired: 3 out]
    n131 = Array Max & Min(array=w191) -> (min value=w196:dbl)  [unwired: 3 out]
    n132 = Array Max & Min(array=w190) -> (min value=w194:dbl)  [unwired: 3 out]
    n133 = Array Max & Min(array=w158) -> (min value=w180:dbl)  [unwired: 3 out]
    n134 = Array Max & Min(array=w159) -> (min value=w178:dbl)  [unwired: 3 out]
    n135 = Array Max & Min(array=w160) -> (min value=w176:dbl)  [unwired: 3 out]
    n136 = Array Max & Min(array=w161) -> (min value=w174:dbl)  [unwired: 3 out]
    n137 = Array Max & Min(array=w162) -> (min value=w206:dbl)  [unwired: 3 out]
    n138 = Array Max & Min(array=w163) -> (min value=w175:dbl)  [unwired: 3 out]
    n139 = Array Max & Min(array=w164) -> (min value=w177:dbl)  [unwired: 3 out]
    n140 = Array Max & Min(array=w165) -> (min value=w179:dbl)  [unwired: 3 out]
    n141 = Array Max & Min(array=w171) -> (min value=w181:dbl)  [unwired: 3 out]
    n142 = Array Max & Min(array=w186) -> (min value=w195:dbl)  [unwired: 3 out]
    n143 = Array Max & Min(array=w187) -> (min value=w197:dbl)  [unwired: 3 out]
    n144 = Array Max & Min(array=w188) -> (min value=w199:dbl)  [unwired: 3 out]
    n145 = Array Max & Min(array=w189) -> (min value=w201:dbl)  [unwired: 3 out]
    n146 = Less?(x=w206, y=3000.0) -> (x < y?=w205:bool)
    n147 = Select(t=w206, s=w205, f=inf) -> (s? t:f=w207:dbl)
    n148 = Build Array(w207, w174, w175, w176, w177, w178, w179, w180, w181, w194, w195, w196, w197, w198, w199, w200, w201) -> (w173:dbl[])
    n149 = Array Max & Min(array=w173) -> (max value=w202:dbl, max index (indices)=w182:i32)  [unwired: 2 out]
    n150 = case shown="1" w182 {
      tunnel: [90.0 95.0 85.0 100.0 80.0 120.0 60.0 130.0 50.0 140.0 40.0 150.0 30.0 160.0 20.0 170.0 10.0] -> w183
      frame 0, Default {
      }
      frame 1 {
      }
      frame 2 {
      }
      frame 3 {
      }
      frame 4 {
      }
      frame 5 {
      }
      frame 6 {
      }
      frame 7 {
      }
      frame 8 {
      }
      frame 9 {
      }
      frame 10 {
      }
      frame 11 {
      }
      frame 12 {
      }
      frame 13 {
      }
      frame 14 {
      }
      frame 15 {
      }
      frame 16 {
      }
    }
    n151 = Less?(x=w202, y="length") -> (x < y?=→"VEstop":bool)
    n152 = Negate(x=w183) -> (-x=w184:dbl)
    n153 = Add(x=90.0, y=w184) -> (x+y=→"Anthena_Steer":dbl)
    n154 = expression code="(x/180.0)*pi" "degrees to radians"(w183) -> (w172:dbl)
    n155 = Polar To Re/Im(2:w172, 3:7000.0 ("r")) -> (0:w167:dbl, 1:w166:dbl)
    n156 = Build Array(w166, w152) -> (w168:dbl[])
    n157 = Build Array(w167, w152) -> (w169:dbl[])
    n158 = Bundle(w168, w169) -> (→"TargetDerection":cluster{dbl[], dbl[]})  [unwired: 1 in]
    n159 = local read "Stop"() -> (w147:bool)
  }
  n160 = flat-sequence {
    frame #0 {
      n161 = local write "InputSteer(cmd)"(0.0 ("InputSteer(cmd)")) -> ()
      n162 = Wait (ms)(milliseconds to wait=u32 1000) -> ()  [unwired: 1 out]
    }
    frame #1 {
      n163 = local write "HLV_Gear"(u8 2 ("HLV_Gear")) -> ()
    }
    frame #2 {
      n164 = while {
        stop <- w368 continue-if-true
        n165 = expression code="x/(0.00001*27*pi*60)"(6.0 ("Input_Spd(kph)")) -> (w371:dbl)
        n166 = local read "NearSteer"() -> (w366:dbl)
        n167 = Negate(x=w366) -> (-x=w367:dbl)
        n168 = expression code="x*4.35*1.8"(w371) -> (w369:dbl)
        n169 = local read "GoBack"() -> (w368:bool)
        n170 = local write "Input_Spd(cmd)"(w367) -> ()
        n171 = local write "Input_Spd(cmd)"(w369) -> ()
      }
    }
    frame #3 {
      w373 = 0.0 ("InputSteer(cmd)")
      n172 = Wait (ms)(milliseconds to wait=u32 1000) -> ()  [unwired: 1 out]
      n173 = local write "InputSteer(cmd)"(w373) -> ()
      n174 = local write "Input_Spd(cmd)"(w373) -> ()
    }
  }
  n175 = VISA Close(VISA resource name=w24, error in (no error)=w23) -> (error out=w25:errorcluster)
  n176 = call <vilib>:"Clear Errors.vi"("error in (no error)"=w25) -> ()  [unwired: 5 in, 2 out]
  n177 = while {
    stop <- w375 stop-if-true
    w378 = -450.0 ("element")
    w380 = 100.0 ("element")
    w379 = 450.0 ("element")
    w401 = 1200.0 ("f")
    w395 = 1200.0 ("element")
    w398 = 0.0 ("element")
    w402 = -300.0 ("element")
    w399 = 800.0 ("element")
    w403 = 100.0 ("element")
    w400 = 450.0 ("element")
    w392 = 0.0 ("element")
    w396 = -300.0 ("element")
    w393 = -800.0 ("element")
    w397 = 100.0 ("element")
    w394 = -450.0 ("element")
    # "뒤로 빠꾸"
    # "가까운 실제 존재 장애물은 피하기"
    # "Neer Steering"
    n178 = local read "X_arraysREAL"() -> (w377:i32[])
    n179 = local read "Y_arraysREAL"() -> (w376:i32[])
    n180 = local read "GoBack"() -> (w374:bool)
    n181 = Select(t=1700.0, s=w374, f=950.0 ("element")) -> (s? t:f=w391:dbl)
    n182 = Build Array(w394, w394, w393, w393, w392, w392, w394) -> (w417:dbl[])
    n183 = Build Array(w397, w396, w396, w395, w395, w397, w397) -> (w416:dbl[])
    n184 = Build Array(w400, w400, w399, w399, w398, w398, w400) -> (w409:dbl[])
    n185 = Build Array(w403, w402, w402, w401, w401, w403, w403) -> (w410:dbl[])
    n186 = Build Array(w379, w379, w378, w378, w379) -> (w388:dbl[])
    n187 = Build Array(w380, w391, w391, w380, w380) -> (w387:dbl[])
    n188 = call "ROI_IN_Check.vi"("도형Y좌표"=w416, "도형X좌표"=w417, "LiDAR_Y"=w376, "LiDAR_X"=w377) -> ("ROI_IN_Y"=w419:i32[], "ROI_IN_X"=w418:i32[])  [unwired: 6 in]
    n189 = Bundle(w417, w416) -> (→"NearCarROILeft":cluster{dbl[], dbl[]})  [unwired: 1 in]
    n190 = call "ROI_IN_Check.vi"("도형Y좌표"=w410, "도형X좌표"=w409, "LiDAR_Y"=w376, "LiDAR_X"=w377) -> ("ROI_IN_Y"=w422:i32[], "ROI_IN_X"=w421:i32[])  [unwired: 6 in]
    n191 = Bundle(w409, w410) -> (→"NearCarROIRight":cluster{dbl[], dbl[]})  [unwired: 1 in]
    n192 = call "ROI_IN_Check.vi"("도형Y좌표"=w387, "도형X좌표"=w388, "LiDAR_Y"=w376, "LiDAR_X"=w377) -> ("ROI_IN_Y"=w384:i32[], "ROI_IN_X"=w385:i32[])  [unwired: 6 in]
    n193 = Bundle(w388, w387) -> (→"GobackROI":cluster{dbl[], dbl[]})  [unwired: 1 in]
    n194 = Bundle("ROI_IN_X"=w418, "ROI_IN_Y"=w419) -> (→"NearCarPointsLeft":cluster{"ROI_IN_X":i32[], "ROI_IN_Y":i32[]})  [unwired: 1 in]
    n195 = Bundle("ROI_IN_X"=w421, "ROI_IN_Y"=w422) -> (→"NearCarPointsRight":cluster{"ROI_IN_X":i32[], "ROI_IN_Y":i32[]})  [unwired: 1 in]
    n196 = Re/Im To Polar(2:w419, 3:w418) -> (1:w420:dbl[])  [unwired: 1 out]
    n197 = Re/Im To Polar(2:w422, 3:w421) -> (1:w423:dbl[])  [unwired: 1 out]
    n198 = Re/Im To Polar(2:w384, 3:w385) -> (1:w383:dbl[])  [unwired: 1 out]
    n199 = Array Max & Min(array=w420) -> (min value=w424:dbl)  [unwired: 3 out]
    n200 = Array Size(array=w420) -> (size(s)=w415:i32)
    n201 = Array Max & Min(array=w423) -> (min value=w425:dbl)  [unwired: 3 out]
    n202 = Array Size(array=w423) -> (size(s)=w408:i32)
    n203 = Array Size(array=w383) -> (size(s)=w389:i32)
    n204 = Divide(x=40000.0, y=w424) -> (x/y=w427:dbl)
    n205 = Not Equal To 0?(x=w415) -> (x != 0?=w432:bool)
    n206 = Divide(x=-40000.0, y=w425) -> (x/y=w429:dbl)
    n207 = Not Equal To 0?(x=w408) -> (x != 0?=w431:bool)
    n208 = Not Equal To 0?(x=w389) -> (x != 0?=w390:bool)
    n209 = Select(t=w427, s=w432, f=0.0) -> (s? t:f=w428:dbl)
    n210 = Select(t=w429, s=w431, f=0.0) -> (s? t:f=w430:dbl)
    n211 = Or(x=w432, y=w431) -> (x .or. y?=→"TooClose":bool)
    n212 = Add(x=w428, y=w430) -> (x+y=→"NearSteer":dbl)
    n213 = local write "GoBack"(w390) -> ()
    n214 = local read "Stop"() -> (w375:bool)
  }
  n215 = Close Python Session(session in=w9, error in=w10) -> (11:→"Clustering Error":errorcluster)
